vi "Close References.vi"(8 "error in":errorcluster, 11 "Data Subject in":refnum<class "Data Subject.lvclass">) -> (0 "error out":errorcluster, 3 "Data Subject out":refnum<class "Data Subject.lvclass">)   [LabVIEW 2015, in "Data Subject.lvclass"]
doc: "Deallocate the memory for the DVR."
uses:
  Data Subject.lvclass
  Data Subject.lvclass/Data Subject.ctl
  Data/Data.lvclass
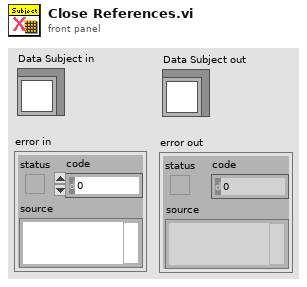
[diagram p1: front panel]
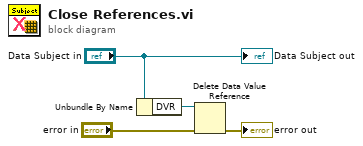
[diagram p0: block diagram]
diagram:
  n1 = Unbundle By Name("Data Subject in") -> ("DVR"=w1:refnum<data-value>)
  n2 = Delete Data Value Reference(data value reference=w1, error in="error in") -> (error out=→"error out":errorcluster)  [unwired: 1 out]
  "Data Subject out" <- "Data Subject in"
